vi "Level Meter.vi"(8 "error in (no error)":errorcluster, 11 "Level Meter in":refnum<class "Level Meter.lvclass">) -> (0 "error out":errorcluster, 3 "Level Meter out":refnum<class "Level Meter.lvclass">)   [LabVIEW 2009, in "Level Meter.lvclass"]
uses:
  Level Meter.lvclass
  Utility Classes/Readable/Channel Names.ctl
  Utility Classes/Readable/Channel Units.ctl
  Oxford/BUSGEN.LLB/OxfordAddress.ctl
  Level Meter.lvclass/Level Meter.ctl
  Utility Classes/Readable/Readable.lvclass
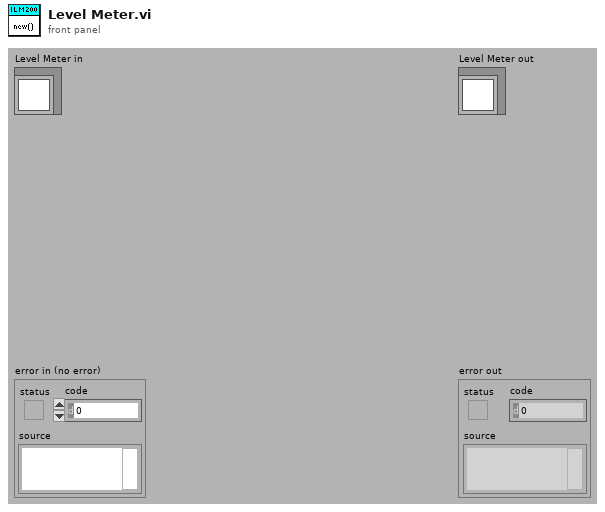
[diagram p1: front panel]
types:
  T1 = typedef "Readable.lvclass/Channel Names.ctl" = string[]
  T2 = typedef "Readable.lvclass/Channel Units.ctl" = string[]
  T3 = typedef "OxfordAddress.ctl" = cluster{"Com Port":i32, "ISOBUS Address":i32, "GPIB Address":i16, "Communication":enum16{"RS232", "ISOBUS", "GPIB", "Gateway"}}
  T4 = cluster{"Address":T3, "ILM Name":string, "Display Channel":i32[]}
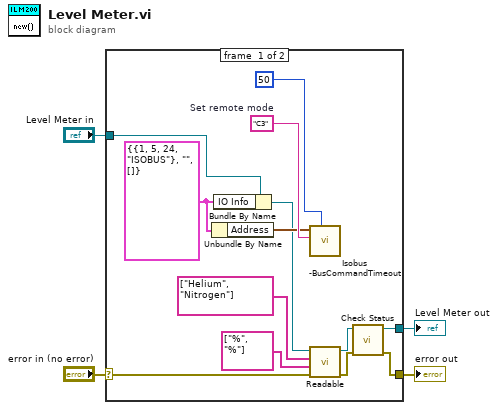
[diagram p0: block diagram]
diagram:
  n1 = case shown="No Error" "error in (no error)" {
    selector: "error in (no error)" -> [w8 w19]
    tunnel: [w5 w19] -> w3
    tunnel: [w7 w18] -> w1
    tunnel: "Level Meter in" -> [w17 w18]
    frame #0 {
      w12 = T4 {"Address"={"Com Port"=1, "ISOBUS Address"=5, "GPIB Address"=24, "Communication"=enum."ISOBUS"}, "ILM Name"="", "Display Channel"=[]} ("ILM Setup")
      w16 = "C3"  # Set remote mode
      n2 = Unbundle By Name(w12) -> ("Address"=w14:T3)
      n3 = Bundle By Name(cluster=w17, "IO Info"=w12) -> (w13:refnum<class "Level Meter.lvclass">)
      n4 = call "Isobus -BusCommandTimeout.vi"("Timeout (ms)"=50, "Command"=w16, "Address"=w14) -> ()  [unwired: 6 out]
      n5 = call "Readable.vi"("error in (no error)"=w8, "Channel Units"=T2 ["%", "%"], "Channel Names"=T1 ["Helium", "Nitrogen"], "Readable in"=w13) -> ("error out"=w6:errorcluster, "Readable out"=w11:refnum<class "Level Meter.lvclass">)  [unwired: 6 in]
      n6 = call-dynamic "Check Status.vi"("error in (no error)"=w6, "Level Meter in"=w11) -> ("error out"=w5:errorcluster, "Level Meter out"=w7:refnum<class "Level Meter.lvclass">)  [unwired: 6 in, 2 out]
    }
    frame #1 {
    }
  }
  "error out" <- w3
  "Level Meter out" <- w1
